vi "new.vi"(6 "taskType":T1(ring), 8 "error in (no error)":errorcluster, 11 "ignoreStopMechanism":bool) -> (0 "error out":errorcluster, 3 "TaskMock out":refnum<class "TaskMock.lvclass">)   [LabVIEW 2023, in "TaskMock.lvclass"]
uses:
  TaskMock.lvclass
  TaskMock.lvclass/TaskMock.ctl
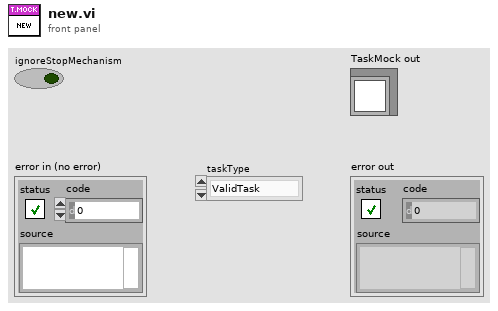
[diagram p1: front panel]
types:
  T1 = enum16{"ValidTask", "BrokenTask", "InvalidConnectorPaneTask"}
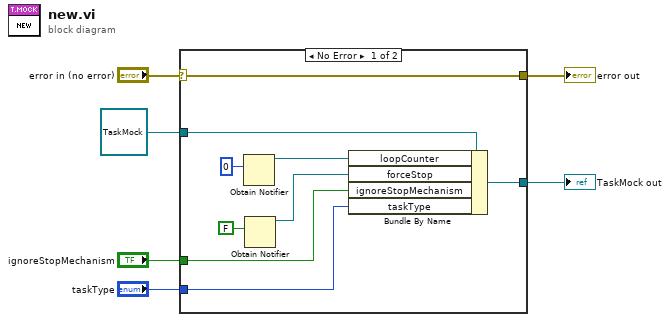
[diagram p0: block diagram]
diagram:
  n1 = case shown="No Error" "error in (no error)" {
    selector: "error in (no error)" -> [w14 w17]
    tunnel: [w14 w17] -> w5
    tunnel: [w12 w16] -> w3
    tunnel: refnum<class "TaskMock.lvclass"> refnum ("TaskMock in") -> [w15 w16]
    tunnel: "ignoreStopMechanism" -> [w8 _]
    tunnel: "taskType" -> [w7 _]
    frame No Error {
      n2 = Obtain Notifier(notification data type=0) -> (notifier out=w11:refnum<notifier>)  [unwired: 3 in, 2 out]
      n3 = Obtain Notifier(notification data type=FALSE) -> (notifier out=w9:refnum<notifier>)  [unwired: 3 in, 2 out]
      n4 = Bundle By Name(cluster=w15, "loopCounter"=w11, "forceStop"=w9, "ignoreStopMechanism"=w8, "taskType"=w7) -> (w12:refnum<class "TaskMock.lvclass">)
    }
    frame Error {
    }
  }
  "error out" <- w5
  "TaskMock out" <- w3
